vi "RT - Initialize States.vi"(8 "error in":errorcluster) -> (0 "error out":errorcluster)   [LabVIEW 2018]
uses:
  Controls/ConfigCalibration.ctl
  Controls/Pumps State.ctl
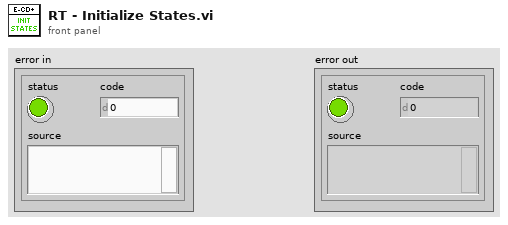
[diagram p1: front panel]
types:
  T1 = typedef "Pumps State.ctl" = enum16{"Do Nothing", "Run Pump 1", "Run Pump 2", "Run Pump 3", "Run Pump 4", "Run Pump 5", "Stop Pump 1", "Stop Pump 2", "Stop Pump 3", "Stop Pump 4", "Stop Pump 5"}
  T2 = typedef "ConfigCalibration.ctl" = enum16{"CAL STOP", "TWTT OP (IN)", "TWTT PDP (IN)", "DLT OP (IN)", "DLT PDP 01 (IN)", "DLT PDP 02 (IN)", "BR OP (IN)", "BR TWT ALIGN (IN)", "BR DL ALIGN (IN)"}
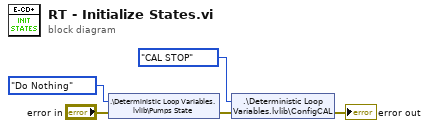
[diagram p0: block diagram]
diagram:
  n1 = shared-variable ".\\Deterministic Loop Variables.lvlib\\Pumps State"(Pumps_State."Do Nothing" ("Pumps State"), error in="error in") -> (error out=w1:errorcluster)
  n2 = shared-variable ".\\Deterministic Loop Variables.lvlib\\ConfigCAL"(ConfigCalibration."CAL STOP" ("ConfigCAL"), error in=w1) -> (error out=→"error out":errorcluster)
